vi "Tiempo_CH3_FGV.vi"(0 "Tiempo_IN":timestamp, 1 "Prox. Estado_IN":bool, 4 "Opción":enum16{"Write", "Read"}(ring), 5 "Error In":errorcluster) -> (14 "Tiempo_OUT":timestamp, 15 "Prox. Estado_OUT":bool, 19 "Error Out":errorcluster)   [LabVIEW 2013]
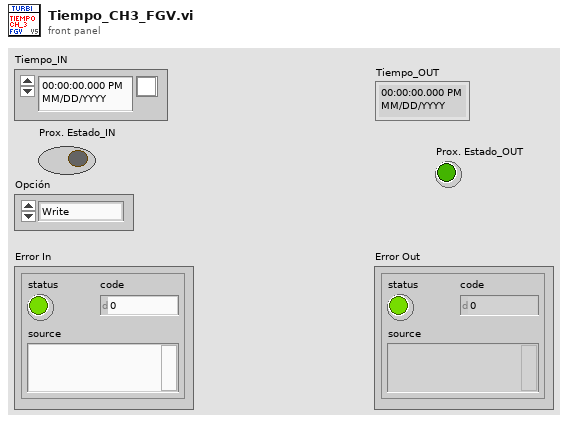
[diagram p1: front panel]
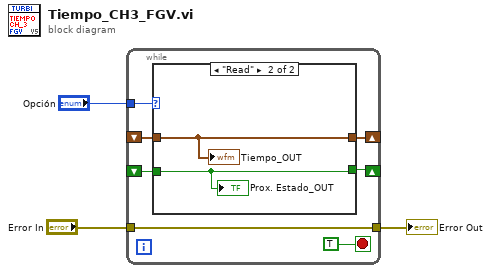
[diagram p0: block diagram]
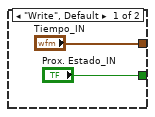
[diagram p2: hidden frame]
diagram:
  n1 = while {
    tunnel: "Opción" -> [w9]
    tunnel: [w8] -> w2
    tunnel: "Error In" -> [w8]
    shift-right: [w7] -> _
    shift-left: _ -> [w6]
    shift-right: [w5] -> _
    shift-left: _ -> [w4]
    stop <- TRUE stop-if-true
    n2 = case shown="\"Read\"" w9 {
      tunnel: ["Tiempo_IN" w14] -> w7
      tunnel: w6 -> [_ w14]
      tunnel: ["Prox. Estado_IN" w13] -> w5
      tunnel: w4 -> [_ w13]
      frame "Write", Default {
      }
      frame "Read" {
        "Tiempo_OUT" <- w14
        "Prox. Estado_OUT" <- w13
      }
    }
  }
  "Error Out" <- w2
